vi "Modifier ParaInst.vi"(1 "Paramètre Instrumentaux Avant":string[][](table)=[["Loral", "10", "100000", "300000", "0", "200000", "4400", "2500", "750000", "1000000", "750000", "1000000"], ["EEV", "10", "250000", "450000", "600000", "1000000", "4200", "2000", "0", "0", "0", "0"], ["Spectro", "10", "400000", "600000", "400000", "600000", "4000", "4500", "0", "0", "0", "0"], ["Panoramix+Loral", "10", "0", "0", "0", "0", "0", "0", "0", "0", "0", "0"], ["Pnoramix+EEV", "10", "0", "0", "0", "0", "0", "0", "0", "0", "0", "0"], ["FantOMM", "10", "0", "0", "0", "0", "0", "0", "0", "0", "0", "0"], ["Monica", "10", "0", "0", "0", "0", "0", "0", "0", "0", "0", "0"], ["Simon", "10", "0", "0", "0", "0", "0", "0", "0", "0", "0", "0"], ["Cpapir", "10", "0", "0", "0", "0", "0", "0", "0", "0", "0", "0"]]) -> (0 "Paramètre Instrumentaux Après":string[][](table)=[["Loral", "10", "100000", "300000", "0", "200000", "4400", "2500", "750000", "1000000", "750000", "1000000"], ["EEV", "10", "250000", "450000", "600000", "1000000", "4200", "2000", "0", "0", "0", "0"], ["Spectro", "10", "400000", "600000", "400000", "600000", "4000", "4500", "0", "0", "0", "0"], ["Panoramix+Loral", "10", "0", "0", "0", "0", "0", "0", "0", "0", "0", "0"], ["Pnoramix+EEV", "10", "0", "0", "0", "0", "0", "0", "0", "0", "0", "0"], ["FantOMM", "10", "0", "0", "0", "0", "0", "0", "0", "0", "0", "0"], ["Monica", "10", "0", "0", "0", "0", "0", "0", "0", "0", "0", "0"], ["Simon", "10", "0", "0", "0", "0", "0", "0", "0", "0", "0", "0"], ["Cpapir", "10", "0", "0", "0", "0", "0", "0", "0", "0", "0", "0"]])   [LabVIEW 2010]
panel:
  in  "Annuler":bool
  in  "Terminer":bool
  in  "Paramètre Instrumentaux":string[][](table)=[["Loral", "10", "100000", "300000", "0", "", "", "", "", "", "", ""], ["EEV", "10", "250000", "450000", "600000", "", "", "", "", "", "", ""], ["Spectro", "10", "400000", "600000", "400000", "", "", "", "", "", "", ""], ["Panoramix+Loral", "10", "0", "0", "0", "", "", "", "", "", "", ""], ["Pnoramix+EEV", "10", "0", "0", "0", "", "", "", "", "", "", ""], ["FantOMM", "10", "0", "0", "0", "", "", "", "", "", "", ""], ["Monica", "10", "0", "0", "0", "", "", "", "", "", "", ""], ["Simon", "10", "0", "0", "0", "", "", "", "", "", "", ""], ["Cpapir", "10", "0", "0", "0", "", "", "", "", "", "", ""]]
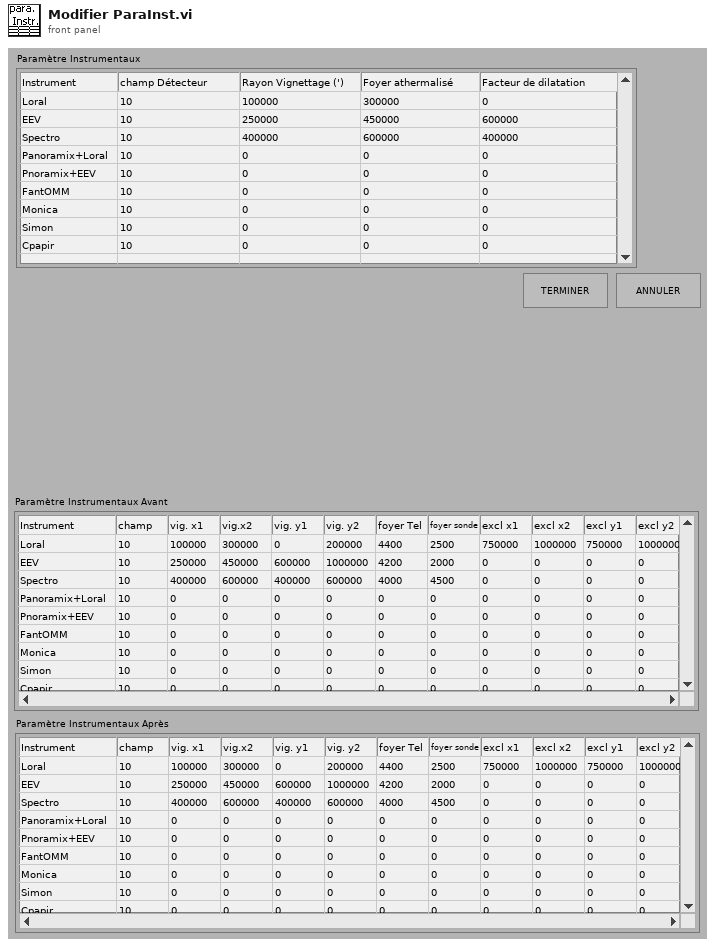
[diagram p1: front panel]
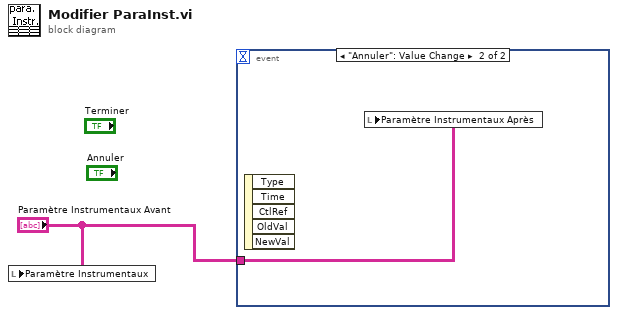
[diagram p0: block diagram]
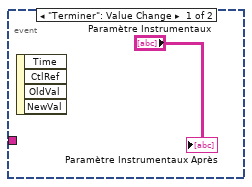
[diagram p2: hidden frame]
diagram:
  n1 = local write "Paramètre Instrumentaux"("Paramètre Instrumentaux Avant") -> ()
  n2 = event shown="[1] \"Annuler\": Value Change" {
    selector: _ -> [_ _]
    dyn-events: _ -> [_ _]
    timeout: _ -> [_ _]
    tunnel: "Paramètre Instrumentaux Avant" -> [_ w3]
    event "Terminer": Value Change {
      n3 = event-data() -> ()  [unwired: 1 in, 4 out]
      "Paramètre Instrumentaux Après" <- "Paramètre Instrumentaux"
    }
    event "Annuler": Value Change {
      n4 = event-data() -> ()  [unwired: 1 in, 5 out]
      n5 = local write "Paramètre Instrumentaux Après"(w3) -> ()
    }
  }
